vi "Timing-Tick Tock.vi"(6 "error in (no error)":errorcluster) -> (1 "Elapsed time (ms)":u32, 2 "error out":errorcluster)   [LabVIEW 2020]
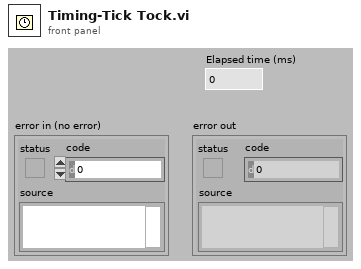
[diagram p1: front panel]
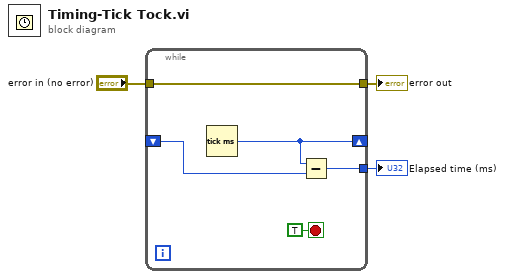
[diagram p0: block diagram]
diagram:
  n1 = while {
    shift-right: [w6] -> _
    shift-left: _ -> [w5]
    tunnel: "error in (no error)" -> [w7]
    tunnel: [w7] -> w2
    tunnel: [w4] -> w1
    stop <- TRUE stop-if-true
    n2 = Tick Count (ms)() -> (millisecond timer value=w6:u32)
    n3 = Subtract(x=w6, y=w5) -> (x-y=w4:u32)
  }
  "error out" <- w2
  "Elapsed time (ms)" <- w1
